vi "1WIRE_RESET.vi"(7 "1-Wire DIO Pin":refnum<k21>="ConnectorA/DIO15", 8 "error in":errorcluster) -> (0 "error out":errorcluster, 1 "0 = Device Present / 1=no":bool)   [LabVIEW 2014]
doc: "This VI is created by Vincent Claes for FPDA-1 more information on http://pwo.fpga.be\n\nvincent.claes@xios.be\nclaesvincent@gmail.com\n\nhttp://www.linkedin.com/in/vincentclaes"
uses:
  <vilib>/rvi/Emulation/niFpgaSctlEmulationGetInTimedLoop.vi
  <vilib>/rvi/Emulation/niFpgaProcessEmulError.vi
  <vilib>/rvi/eio/common/nirviEmuTemplateMethod_errors.vi
  <vilib>/eio/EIOMethodNode/EIOMethodNode.xnode
  <vilib>/eio/EIONode/EIONode.xnode
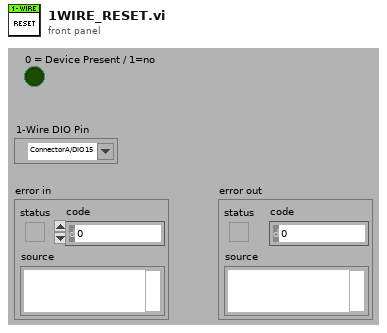
[diagram p1: front panel]
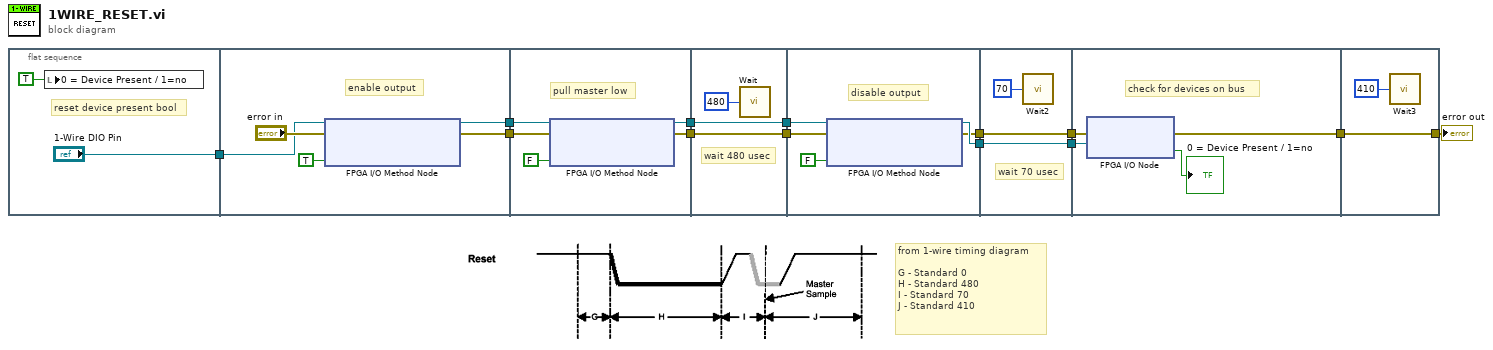
[diagram p0: block diagram]
diagram:
  # "from 1-wire timing diagram\n\nG - Standard 0\nH - Standard 480\nI - Standard 70\nJ - Standard 410"
  n1 = flat-sequence {
    tunnel: ["1-Wire DIO Pin"] -> w1
    tunnel: [w19] -> w13
    tunnel: [w18] -> w12
    tunnel: w1 -> [w16]
    tunnel: w13 -> [w25]
    tunnel: w12 -> [w24]
    tunnel: [w23] -> w4
    tunnel: [w22] -> w3
    tunnel: [w27] -> w5
    tunnel: w4 -> [w27]
    tunnel: w3 -> [w26]
    tunnel: [w26] -> w2
    tunnel: [w32] -> w11
    tunnel: [w31] -> w10
    tunnel: w5 -> [w30]
    tunnel: w2 -> [w29]
    tunnel: [w35] -> w9
    tunnel: w11 -> [w35]
    tunnel: w10 -> [w34]
    tunnel: [w34] -> w8
    tunnel: w9 -> [w39]
    tunnel: w8 -> [w38]
    tunnel: [w37] -> w7
    tunnel: w7 -> [w41]
    tunnel: [w41] -> w6
    frame #0 {
      # "reset device present bool"
      n2 = local write "0 = Device Present / 1=no"(TRUE ("0 = Device Present / 1=no")) -> ()
    }
    frame #1 {
      # "enable output"
      n3 = xnode "FPGA I/O Method Node"("error in"="error in", "FPGA I/O In"=w16, "Enable"=TRUE ("Data")) -> ("error out"=w18:errorcluster, "FPGA I/O Out"=w19:refnum<k21>)
    }
    frame #2 {
      # "pull master low"
      n4 = xnode "FPGA I/O Method Node"("error in"=w24, "FPGA I/O In"=w25, "Data"=FALSE ("FX2_IO1_J1_0")) -> ("error out"=w22:errorcluster, "FPGA I/O Out"=w23:refnum<k21>)
    }
    frame #3 {
      # "wait 480 usec"
      n5 = call "Wait"("Count(uSec)"=u32 480) -> ()  [unwired: 1 out]
    }
    frame #4 {
      # "disable output"
      n6 = xnode "FPGA I/O Method Node"("error in"=w29, "FPGA I/O In"=w30, "Enable"=FALSE ("Data")) -> ("error out"=w31:errorcluster, "FPGA I/O Out"=w32:refnum<k21>)
    }
    frame #5 {
      # "wait 70 usec"
      n7 = call "Wait2"("Count(uSec)"=u32 70) -> ()  [unwired: 1 out]
    }
    frame #6 {
      # "check for devices on bus"
      n8 = xnode "FPGA I/O Node"("error in"=w38, "FPGA I/O In"=w39) -> ("error out"=w37:errorcluster, "I/O Item"=→"0 = Device Present / 1=no":bool)  [unwired: 1 out]
    }
    frame #7 {
      n9 = call "Wait3"("Count(uSec)"=u32 410) -> ()  [unwired: 1 out]
    }
  }
  "error out" <- w6
